vi "Image Processing.vi"() -> ()   [LabVIEW 2018]
uses:
  <vilib>/Platform/TimedLoop/XDataNode/timing_clust.ctl
  <vilib>/Platform/TimedLoop/XDataNode/nitl_modes.ctl
  <vilib>/Platform/TimedLoop/XDataNode/wakeup.ctl
  <extravilib>/ChannelInstances/Tag-a[.](dbl)/Read With Abort.vi
  <extravilib>/ChannelInstances/Tag-bool/Write With Abort.vi
  <extravilib>/ChannelInstances/Tag-bool/Read With Abort.vi
  <extravilib>/ChannelInstances/Tag-a[.](dbl)/Write With Abort.vi
  <extravilib>/ChannelInstances/Tag-bool/Instantiate.vi
  <extravilib>/ChannelInstances/Tag-a[.](dbl)/Instantiate.vi
  <extravilib>/ChannelInstances/Tag-a[.](dbl)/EndpointRead.vi
  <extravilib>/ChannelInstances/Tag-bool/Endpoint.vi
  <extravilib>/ChannelInstances/Tag-bool/EndpointRead.vi
  <extravilib>/ChannelInstances/Tag-a[.](dbl)/Endpoint.vi
  <vilib>/Platform/TimedLoop/XDataNode/XDataNode.xnode
  <extravilib>/ChannelInstances/Tag-bool.lvlib
  <extravilib>/ChannelInstances/Tag-a[.](dbl).lvlib
  <vilib>/vision/NI_Vision_Development_Module.lvlib
  <vilib>/Platform/TimedLoop/XDataNode/XDNodeRunTimeDep.lvlib
panel:
  out "Template \nImage":T1(plugin-control)
  in  "Minimum \nMatch Score":sgl=500.0
  in  "Grayscale Threshold":cluster{sgl, sgl}(slide)={0.0, 21.377245} scale=0.0..255.0
  out "Grayscale Threshold":T1(plugin-control)
  out "School Detected":bool
  out "Traffic":bool=TRUE
  in  "Luminance Threshold":cluster{i32, i32}(slide)={0, 81} scale=0.0..255.0
  in  "Saturation Threshold":cluster{i32, i32}(slide)={0, 90} scale=0.0..255.0
  in  "Hue Threshold":cluster{i32, i32}(slide)={150, 255} scale=0.0..255.0
  in  "Stop Button":bool
  out "Calibrated":bool=TRUE
  out "Source image":T1(plugin-control)
  out "Masked HSL Threshold":T1(plugin-control)
  out "# of Matches":i32
  out "HSL Threshold":T1(plugin-control)
  in  "Enable Motion":bool=TRUE
  # "Mechatronic Systems Board"
  # "Image Processing"
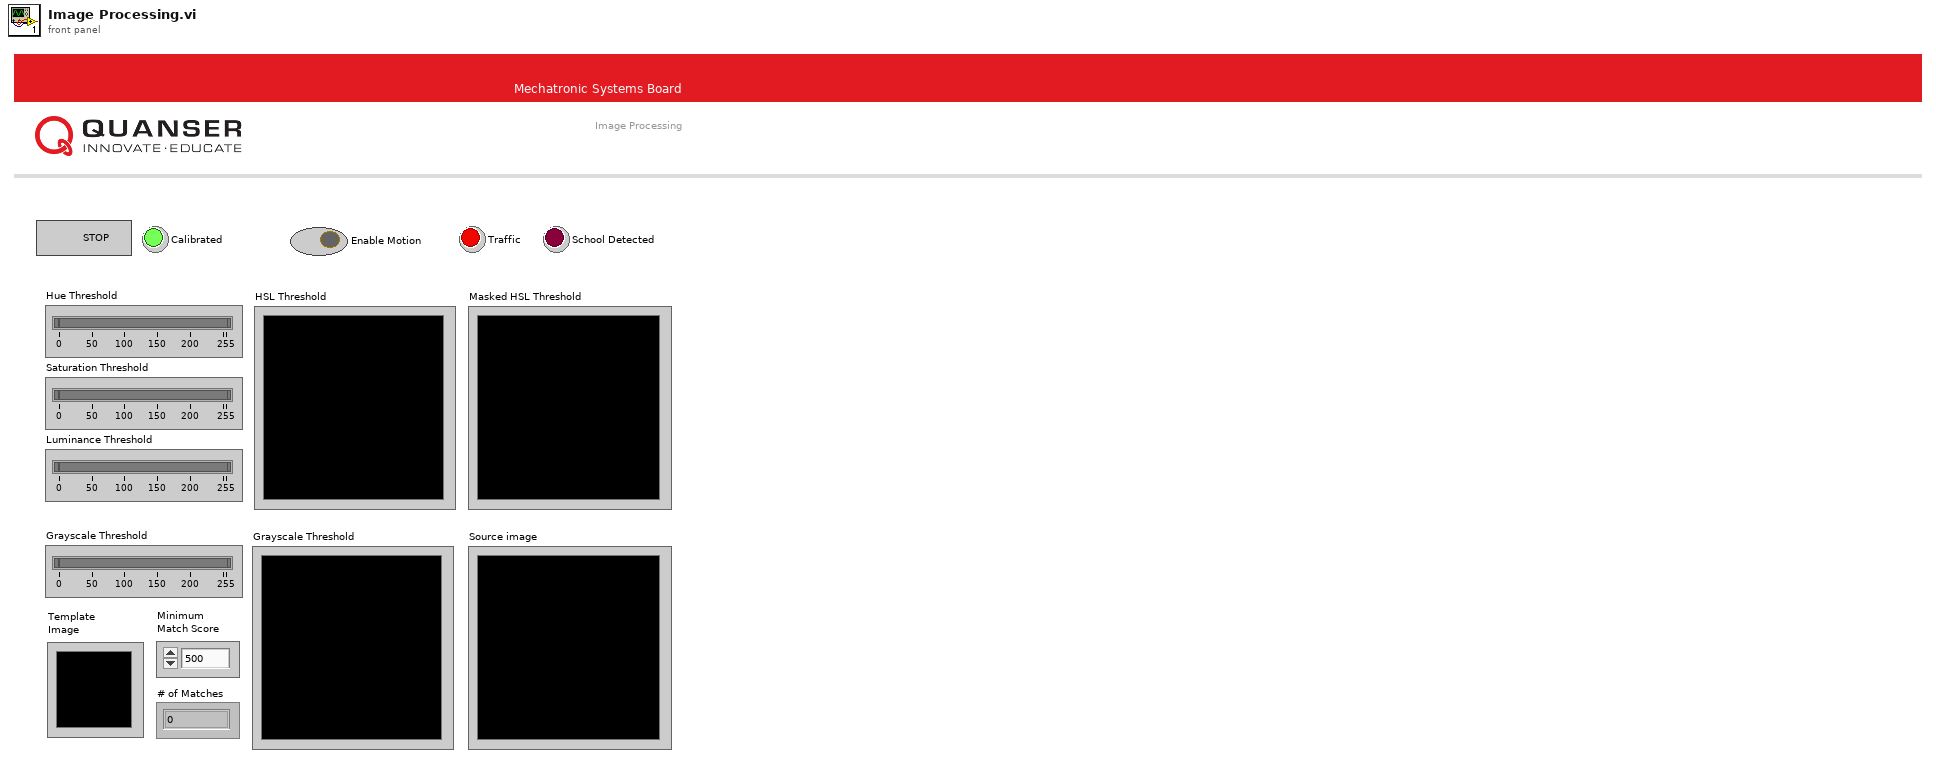
[diagram p1: front panel]
types:
  T1 = typedef "IMAQ Image.ctl" = refnum<image>
  T2 = typedef "QNET MS IO Cluster.ctl" = cluster{"Error":errorcluster, "Encoder Calibration Values":i32[], "Update Calibration":bool, "JPEG Resolutions":u16, "Raw Resolutions":u16, "Image Mode":enum16{"RAW RGB", "RAW Gray Scale", "JPEG"}, "FPGA Ref":refnum<k20>}
  T3 = typedef "XDNodeRunTimeDep.lvlib/timing_clust.ctl" = cluster{"Expected End [f-1]":u64, "Actual End [f-1]":u64, "Finished Late? [f-1]":bool, "Expected End [i-1]":u64, "Actual End [i-1]":u64, "Finished Late? [i-1]":bool, "Expected Start [i]":u64, "Actual Start [i]":u64, "Expected Start [f]":u64, "Actual Start [f]":u64, "Source Name":string, "Structure Name":string, "Period":i64, "Deadline":i64, "Offset":i64, "Start":i64, "Priority":i32, "Timeout":i32, "Mode":T4, "Wakeup Reason":T5, "Error":errorcluster, "Source Type":string, "Secondary Source Type":string, "Global End Time":u64, "Global Start Time":u64, "Frame Duration":u64, "Iteration Duration":u64, "Assigned CPU":i32, "I/O Scan Engine Mode":u32}
  T4 = typedef "XDNodeRunTimeDep.lvlib/nitl_modes.ctl" = enum32{"No Change", "Process missed periods, maintain original phase", "Discard missed periods, maintain original phase", "Process missed periods, ignore original phase", "Discard missed periods, ignore original phase"}
  T5 = typedef "XDNodeRunTimeDep.lvlib/wakeup.ctl" = enum32{"Normal", "Aborted", "Asynchronous wakeup", "Timing source error", "Timed loop error", "Timeout"}
  T6 = cluster{"Algorithm":i32, "Number of Matches Requested":i32, "Minimum Match Score":sgl, "SubPixel Accuracy":bool, "Rotation Angle Ranges":cluster{"Start":sgl, "End":sgl}[], "Show Search Area":bool, "Show Result":bool}
  T7 = typedef "ROI Descriptor" = cluster{"Global Rectangle":i32[], "Contours":cluster{"ID":enum32{"External", "Internal"}, "Type":u32, "Coordinates":i32[]}[]}
  T8 = cluster{"Area":dbl, "Number of Holes":dbl, "Bounding Rect":cluster{"Left":dbl, "Top":dbl, "Right":dbl, "Bottom":dbl}, "Center of Mass":cluster{"X":dbl, "Y":dbl}, "Orientation":dbl, "Dimensions":cluster{"Width":dbl, "Height":dbl}}[]
  T9 = typedef "Tag-bool.lvlib/))Channel.ctl" = refnum<queue>
  T10 = typedef "Tag-a[.](dbl).lvlib/))Channel.ctl" = refnum<queue>
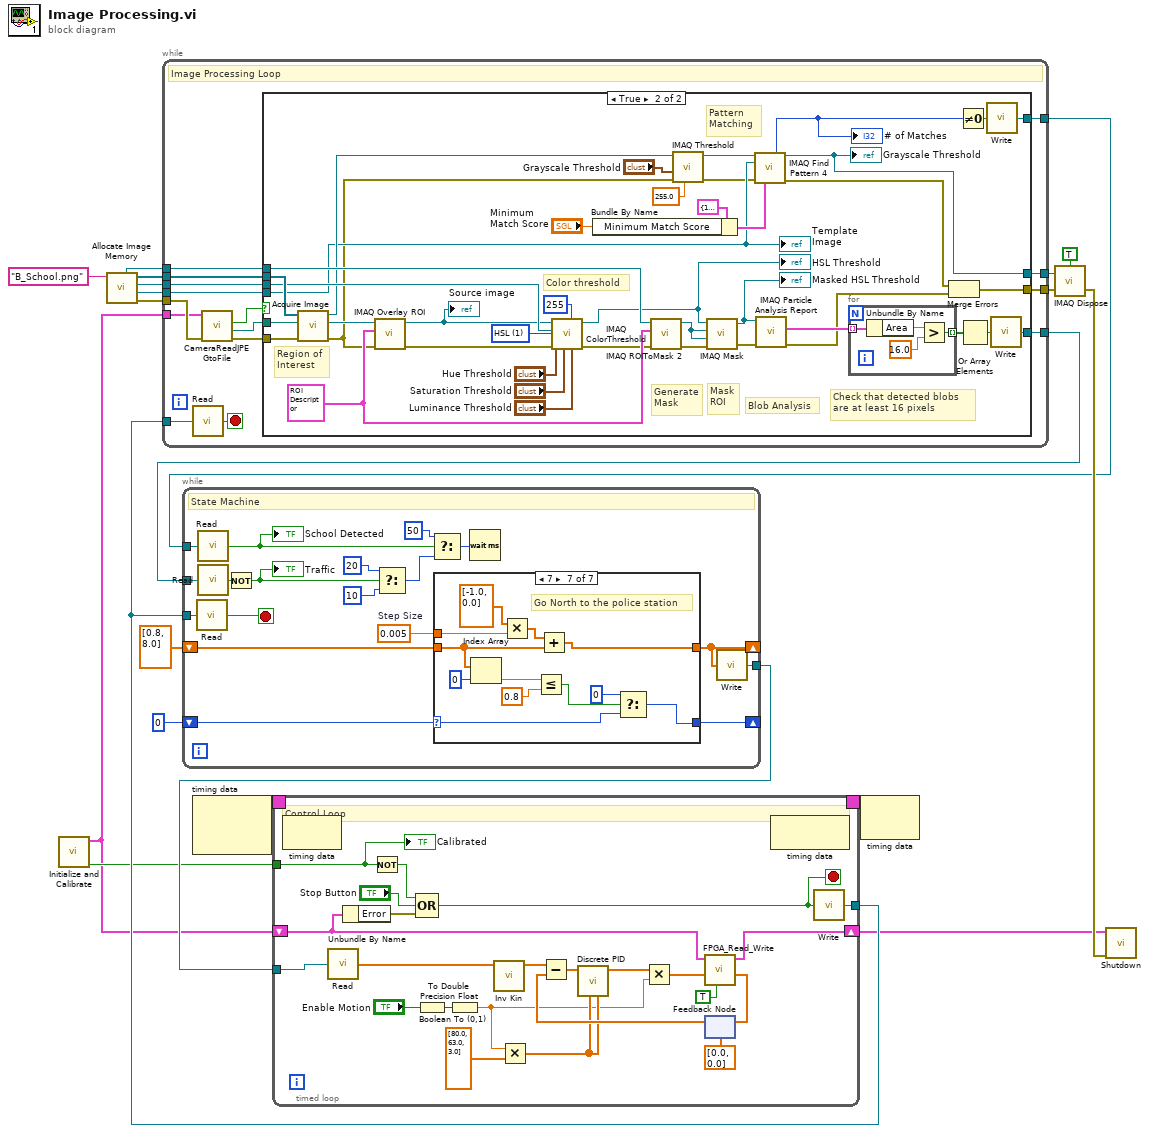
[diagram p0: block diagram]
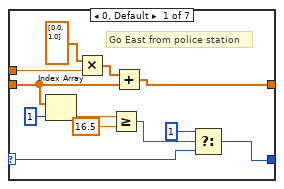
[diagram p3: hidden frame]
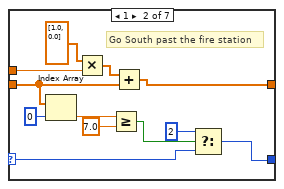
[diagram p4: hidden frame]
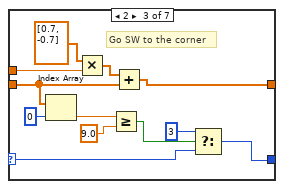
[diagram p5: hidden frame]
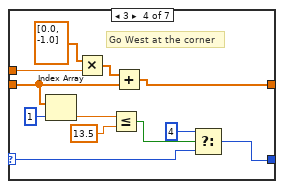
[diagram p6: hidden frame]
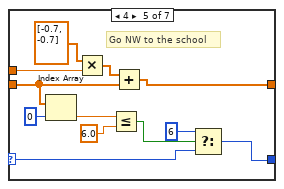
[diagram p7: hidden frame]
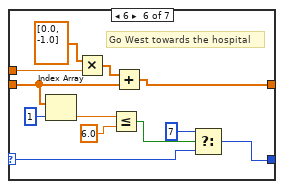
[diagram p8: hidden frame]
diagram:
  n1 = call "Initialize and Calibrate.vi"() -> ("Calibrated"=w8:bool, "IO Cluster"=w7:T2)  [unwired: 10 in]
  n2 = call "Allocate Image Memory.vi"("Reference Image File"="B_School.png") -> ("error out"=w15:errorcluster, "Reference Image"=w16:T1, "HSL Threshold"=w14:T1, "Acquisition Memory"=w17:T1[], "Mask"=w4:T1)  [unwired: 5 in, 1 out]
  n3 = node-c288() -> (w13:T3)  [unwired: 2 in]
  n4 = while {
    tunnel: [w36] -> w20
    tunnel: [w34] -> w18
    tunnel: w17 -> [w31]
    tunnel: w16 -> [w29]
    tunnel: w15 -> [w30]
    tunnel: w14 -> [w28]
    tunnel: w7 -> [w27]
    tunnel: w9 -> [w26]
    tunnel: [w24] -> w11
    tunnel: w4 -> [w23]
    tunnel: [w22] -> w3
    stop <- w25 stop-if-true
    # "Image Processing Loop"
    n5 = call <extravilib>:"Read.vi"("channel"=w26) -> ("element"=w25:bool)  [unwired: 1 in, 1 out]
    n6 = call "CameraReadJPEGtoFile.vi"("error in"=w30, "IO Cluster In"=w27) -> ("Error Out"=w32:errorcluster, "Image File"=w35:path, "New Image Data"=w33:bool)  [unwired: 6 in, 1 out]
    n7 = case shown="True" w33 {
      tunnel: [w38 w41] -> w36
      tunnel: w35 -> [_ w74]
      tunnel: [w37 w40] -> w34
      tunnel: w32 -> [w38 w73]
      tunnel: w31 -> [_ w75]
      tunnel: w29 -> [_ w48]
      tunnel: w28 -> [w37 w72]
      tunnel: [_ w70] -> w24
      tunnel: w23 -> [_ w57]
      tunnel: [_ w45] -> w22
      frame False {
      }
      frame True {
        w39 = u16 1 items=["RGB", "HSL", "HSV", "HSI"] ("Color Mode")
        w64 = T7 {"Global Rectangle"=[48, 48, 80, 80], "Contours"=[{"ID"=enum."Internal", "Type"=3, "Coordinates"=[48, 48, 80, 80]}]} ("ROI Descriptor")
        # "Mask\nROI"
        # "Region of\nInterest"
        # "Generate\nMask"
        # "Pattern\nMatching"
        # "Check that detected blobs \nare at least 16 pixels"
        # "Color threshold"
        # "Blob Analysis"
        n8 = call "Acquire Image.vi"("Error In"=w73, "File Path"=w74, "Acquisition Memory"=w75) -> ("Error Out"=w46:errorcluster, "HSL Image"=w66:T1, "Pre-processed Image"=w56:T1)  [unwired: 4 in, 2 out]
        n9 = call "IMAQ Overlay ROI"("error in (no error)"=w46, "ROI Descriptor"=w64, "Image"=w66) -> ("error out"=w63:errorcluster, "Image Out"=w65:T1)  [unwired: 7 in]
        "Source image" <- w65
        n10 = call "IMAQ ColorThreshold"("Blue or Luma or Val or Inten Range"="Luminance Threshold", "Replace Value"=255, "Green or Sat Range"="Saturation Threshold", "Color Mode"=w39, "error in (no error)"=w63, "Red or Hue Range"="Hue Threshold", "Image Dst"=w72, "Image Src"=w65) -> ("error out"=w47:errorcluster, "Image Dst Out"=w54:T1)  [unwired: 2 in]
        "HSL Threshold" <- w54
        n11 = Bundle By Name(cluster=T6 {"Algorithm"=1, "Number of Matches Requested"=1, "Minimum Match Score"=800.0, "SubPixel Accuracy"=TRUE, "Rotation Angle Ranges"=[], "Show Search Area"=FALSE, "Show Result"=TRUE} ("Settings"), "Minimum Match Score"="Minimum \nMatch Score") -> (w49:T6)
        n12 = call "IMAQ ROIToMask 2"("error in (no error)"=w47, "ROI Descriptor"=w64, "Image"=w57) -> ("error out"=w59:errorcluster, "Image Out"=w62:T1)  [unwired: 6 in, 1 out]
        n13 = call "IMAQ Threshold"("Replace Value"=sgl 255.0, "error in (no error)"=w46, "Range"="Grayscale Threshold", "Image Src"=w56) -> ("error out"=w44:errorcluster, "Image Dst Out"=w55:T1)  [unwired: 6 in]
        n14 = call "IMAQ Mask"("error in (no error)"=w59, "Image Dst"=w62, "Image Mask"=w62, "Image Src"=w54) -> ("error out"=w60:errorcluster, "Image Dst Out"=w61:T1)  [unwired: 1 in]
        "Masked HSL Threshold" <- w61
        n15 = call "IMAQ Find Pattern 4"("Image"=w55, "Template"=w48, "error in"=w44, "Settings"=w49) -> ("Number of Matches"=w58:i32, "Image Out"=w40:T1, "error out"=w43:errorcluster)  [unwired: 5 in, 4 out]
        "# of Matches" <- w58
        "Grayscale Threshold" <- w40
        n16 = call "IMAQ Particle Analysis Report"("error in (no error)"=w60, "Image"=w61) -> ("error out"=w42:errorcluster, "Particle Reports (Pixels)"=w69:T8)  [unwired: 4 in, 4 out]
        n17 = for {
          tunnel: w69 -> [w83] mode=indexing
          tunnel: [w80] -> w68 mode=indexing
          n18 = Unbundle By Name(w83) -> ("Area"=w82:dbl)
          n19 = Greater?(x=w82, y=16.0) -> (0:w80:bool)
        }
        n20 = Merge Errors(w43, w42) -> (w41:errorcluster)
        n21 = Not Equal To 0?(x=w58) -> (x != 0?=w71:bool)
        n22 = Or Array Elements(Boolean array=w68) -> (logical OR=w67:bool)
        n23 = call <extravilib>:"Write.vi"("element"=w71) -> ("channel"=w45:T9)  [unwired: 1 out]
        n24 = call <extravilib>:"Write.vi"("element"=w67) -> ("channel"=w70:T9)  [unwired: 1 out]
        "Template \nImage" <- w48
      }
    }
  }
  n25 = call "IMAQ Dispose"("All Images? (No)"=TRUE, "Image"=w18, "error in (no error)"=w20) -> ("error out"=w21:errorcluster)  [unwired: 3 in]
  n26 = while {
    tunnel: [w101] -> w10
    tunnel: w9 -> [w100]
    tunnel: w11 -> [w98]
    tunnel: w3 -> [w97]
    shift-right: [w87] -> _
    shift-left: u32 0 ("millisecond multiple") -> [w90]
    shift-right: [w86] -> _
    shift-left: dbl[] [0.8, 8.0] ("appended array") -> [w89]
    stop <- w99 stop-if-true
    w88 = 0.005  # Step Size
    # "State Machine"
    n27 = call <extravilib>:"Read.vi"("channel"=w100) -> ("element"=w99:bool)  [unwired: 1 in, 1 out]
    n28 = call <extravilib>:"Read.vi"("channel"=w97) -> ("element"=w91:bool)  [unwired: 1 in, 1 out]
    "School Detected" <- w91
    n29 = call <extravilib>:"Read.vi"("channel"=w98) -> ("element"=w85:bool)  [unwired: 1 in, 1 out]
    n30 = Not(x=w85) -> (.not. x?=w84:bool)
    "Traffic" <- w84
    n31 = Select(t=u32 20, s=w84, f=u32 10 ("millisecond multiple")) -> (s? t:f=w92:u32)
    n32 = Select(t=u32 50 ("millisecond multiple"), s=w91, f=w92) -> (s? t:f=w95:u32)
    n33 = case shown="7" w90 {
      selector: w90 -> [w104 w116 w128 w140 w152 w164 w176]
      tunnel: w89 -> [w108 w120 w132 w144 w156 w168 w180]
      tunnel: [w110 w122 w134 w146 w158 w170 w182] -> w86
      tunnel: w88 -> [w112 w124 w136 w148 w160 w172 w184]
      tunnel: [w103 w115 w127 w139 w151 w163 w175] -> w87
      frame 0, Default {
        # "Go East from police station"
        n34 = Index Array(array=w108, index=1) -> (element=w107:dbl)
        n35 = Multiply(x=dbl[] [0.0, 1.0] ("appended array"), y=w112) -> (x*y=w113:dbl[])
        n36 = Greater Or Equal?(x=w107, y=16.5) -> (x >= y?=w105:bool)
        n37 = Add(x=w113, y=w108) -> (x+y=w110:dbl[])
        n38 = Select(t=u32 1, s=w105, f=w104) -> (s? t:f=w103:u32)
      }
      frame 1 {
        # "Go South past the fire station"
        n39 = Index Array(array=w120, index=0) -> (element=w119:dbl)
        n40 = Multiply(x=dbl[] [1.0, 0.0] ("appended array"), y=w124) -> (x*y=w125:dbl[])
        n41 = Greater Or Equal?(x=w119, y=7.0) -> (x >= y?=w117:bool)
        n42 = Add(x=w125, y=w120) -> (x+y=w122:dbl[])
        n43 = Select(t=u32 2, s=w117, f=w116) -> (s? t:f=w115:u32)
      }
      frame 2 {
        # "Go SW to the corner"
        n44 = Index Array(array=w132, index=0) -> (element=w131:dbl)
        n45 = Multiply(x=dbl[] [0.7, -0.7] ("appended array"), y=w136) -> (x*y=w137:dbl[])
        n46 = Greater Or Equal?(x=w131, y=9.0) -> (x >= y?=w129:bool)
        n47 = Add(x=w137, y=w132) -> (x+y=w134:dbl[])
        n48 = Select(t=u32 3, s=w129, f=w128) -> (s? t:f=w127:u32)
      }
      frame 3 {
        # "Go West at the corner"
        n49 = Index Array(array=w144, index=1) -> (element=w143:dbl)
        n50 = Multiply(x=dbl[] [0.0, -1.0] ("appended array"), y=w148) -> (x*y=w149:dbl[])
        n51 = Less Or Equal?(x=w143, y=13.5) -> (x <= y?=w141:bool)
        n52 = Add(x=w149, y=w144) -> (x+y=w146:dbl[])
        n53 = Select(t=u32 4, s=w141, f=w140) -> (s? t:f=w139:u32)
      }
      frame 4 {
        # "Go NW to the school"
        n54 = Index Array(array=w156, index=0) -> (element=w155:dbl)
        n55 = Multiply(x=dbl[] [-0.7, -0.7] ("appended array"), y=w160) -> (x*y=w161:dbl[])
        n56 = Less Or Equal?(x=w155, y=6.0) -> (x <= y?=w153:bool)
        n57 = Add(x=w161, y=w156) -> (x+y=w158:dbl[])
        n58 = Select(t=u32 6, s=w153, f=w152) -> (s? t:f=w151:u32)
      }
      frame 6 {
        # "Go West towards the hospital"
        n59 = Index Array(array=w168, index=1) -> (element=w167:dbl)
        n60 = Multiply(x=dbl[] [0.0, -1.0] ("appended array"), y=w172) -> (x*y=w173:dbl[])
        n61 = Less Or Equal?(x=w167, y=6.0) -> (x <= y?=w165:bool)
        n62 = Add(x=w173, y=w168) -> (x+y=w170:dbl[])
        n63 = Select(t=u32 7, s=w165, f=w164) -> (s? t:f=w163:u32)
      }
      frame 7 {
        # "Go North to the police station"
        n64 = Index Array(array=w180, index=0) -> (element=w179:dbl)
        n65 = Multiply(x=dbl[] [-1.0, 0.0] ("appended array"), y=w184) -> (x*y=w185:dbl[])
        n66 = Less Or Equal?(x=w179, y=0.8) -> (x <= y?=w177:bool)
        n67 = Add(x=w185, y=w180) -> (x+y=w182:dbl[])
        n68 = Select(t=u32 0, s=w177, f=w176) -> (s? t:f=w175:u32)
      }
    }
    n69 = Wait (ms)(milliseconds to wait=w95) -> ()  [unwired: 1 out]
    n70 = call <extravilib>:"Write.vi"("element"=w86) -> ("channel"=w101:T10)  [unwired: 1 out]
  }
  n71 = timed-loop {
    timing: w13 -> [_]
    timing-out: [_] -> w12
    shift-right: [w199] -> w6
    shift-left: w7 -> [w200]
    tunnel: w8 -> [w206]
    tunnel: w10 -> [w204]
    tunnel: [w193] -> w9
    stop <- w194 stop-if-true
    # "Control Loop"
    n72 = node-c288() -> ()  [unwired: 1 in, 1 out]
    n73 = call <extravilib>:"Read.vi"("channel"=w204) -> ("element"=w203:dbl[])  [unwired: 1 in, 1 out]
    n74 = Unbundle By Name(w200) -> ("Error"=w205:errorcluster)
    n75 = Not(x=w206) -> (.not. x?=w207:bool)
    n76 = Compound Arithmetic op=OR(w207, "Stop Button", w205) -> (w194:bool)
    n77 = Boolean To (0,1)(Boolean="Enable Motion") -> (0, 1=w189:i16)
    n78 = To Double Precision Float(number=w189) -> (double precision float=w186:dbl)
    n79 = call "Inv Kin.vi"("Task Coordinates (cm)"=w203) -> ("Joint Coordinates (rad)"=w202:dbl[])  [unwired: 10 in]
    n80 = Multiply(x=w186, y=dbl[] [80.0, 63.0, 3.0] ("Joint Coordinates (rad)")) -> (x*y=w190:dbl[])
    n81 = feedback #1(dbl[] [0.0, 0.0] ("Joint Coordinates (rad)")) -> (w197:dbl[])
    n82 = Subtract(x=w202, y=w197) -> (x-y=w201:dbl[])
    n83 = call "Discrete PID.vi"("Gains Motor 1"=w190, "Gains Motor 0"=w190, "Error Array"=w201) -> ("Voltage"=w188:dbl[])  [unwired: 8 in]
    n84 = Multiply(x=w188, y=w186) -> (x*y=w187:dbl[])
    n85 = call "FPGA_Read_Write.vi"("Motors enabled?"=TRUE, "Commands"=w187, "IO Cluster In"=w200) -> ("Joint Coordinates (rad)"=w198:dbl[], "IO Cluster Out"=w199:T2)  [unwired: 5 in, 2 out]
    n86 = feedback-in #1(w198) -> ()
    n87 = node-c288() -> ()  [unwired: 1 in, 1 out]
    n88 = call <extravilib>:"Write.vi"("element"=w194) -> ("channel"=w193:T9)  [unwired: 1 out]
    "Calibrated" <- w206
  }
  n89 = node-c288(w12) -> ()  [unwired: 1 out]
  n90 = call "Shutdown.vi"("Image Processing Loop"=w21, "IO Cluster In"=w6) -> ()  [unwired: 9 in, 1 out]
